vi "Project Open VI Tester.vi"(8 "error in (no error)":errorcluster, 11 "application reference (This Application)":refnum<vi>) -> (0 "error out":errorcluster)   [LabVIEW 2011, in "VI Tester Project API.lvlib"]
uses:
  VI Tester Project API.lvlib
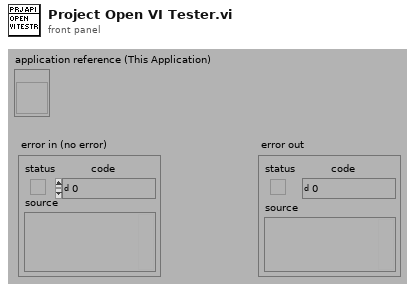
[diagram p1: front panel]
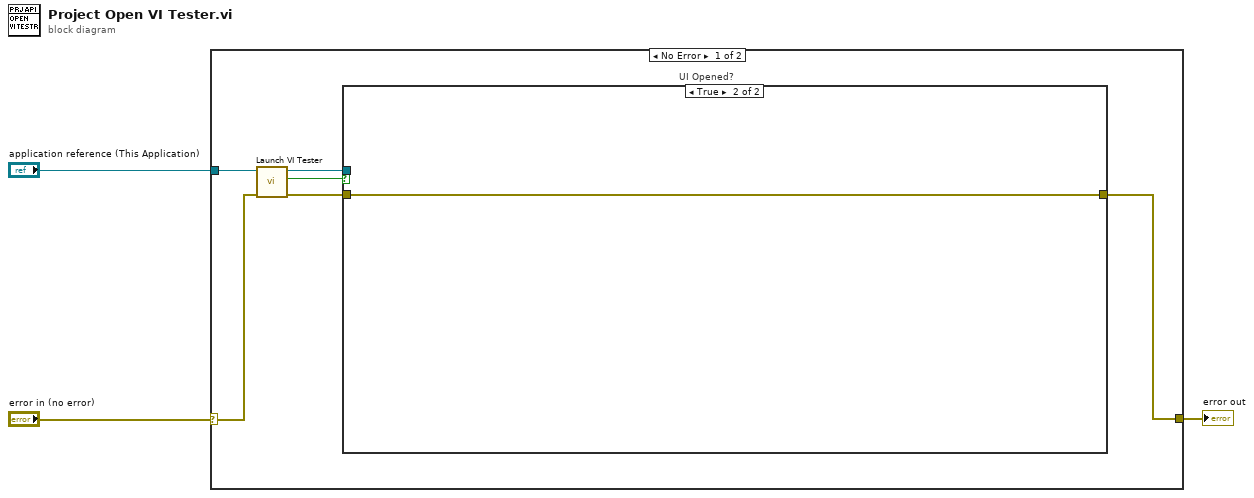
[diagram p0: block diagram]
diagram:
  n1 = case shown="No Error" "error in (no error)" {
    selector: "error in (no error)" -> [w4 w12]
    tunnel: "application reference (This Application)" -> [w5 _]
    tunnel: [w7 w12] -> w2
    frame No Error {
      n2 = call "Launch VI Tester.vi"("error in (no error)"=w4, "application reference"=w5) -> ("error out"=w9:errorcluster, "Opened UI?"=w8:bool, "VI Tester Ref"=w6:refnum<vi>)  [unwired: 7 in]
      n3 = case "UI Opened?" shown="True" w8 {
        tunnel: w9 -> [w10 w11]
        tunnel: [w10 w11] -> w7
        tunnel: w6 -> [_ _]
        frame False {
          # "UI Already open or error"
        }
        frame True {
        }
      }
    }
    frame Error {
    }
  }
  "error out" <- w2
